vi "Check for Included Angle in Degrees.vi"(5 "coerce output (F)":bool, 7 "output range (-180 to 180)":T1=enum."-180 to 180", 9 "right angle (deg)":dbl, 10 "target angle (deg)":dbl, 11 "left angle (deg)":dbl) -> (1 "in range?":bool, 2 "target angle out (deg)":dbl)   [LabVIEW 2017, in "NI_Robotics Utilities.lvlib"]
doc: "This VI is deprecated. Use <vi.lib>\\Analysis\\coordinate.llb\\Check for Included Angle.vi instead."
uses:
  <vilib>/robotics/Utilities/NI_Robotics Utilities.lvlib
  <vilib>/robotics/Utilities/Angle Range_Degrees.ctl
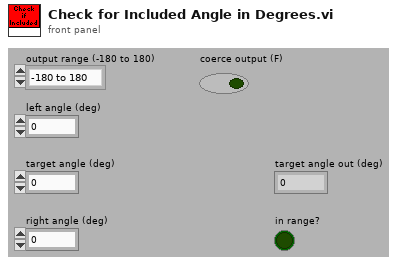
[diagram p1: front panel]
types:
  T1 = typedef "NI_Robotics Utilities.lvlib/Angle Range_Degrees.ctl" = enum16{"none", "-180 to 180", "0 to 360"}
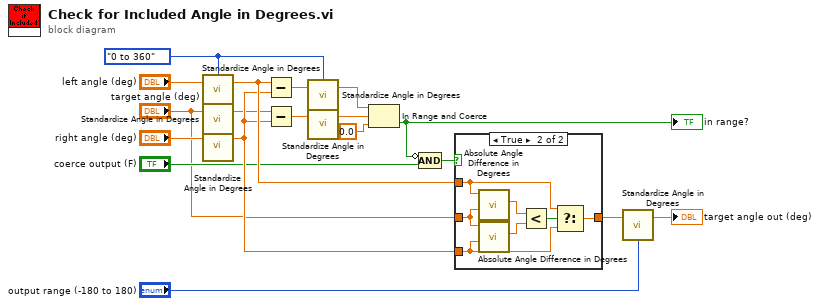
[diagram p0: block diagram]
diagram:
  w13 = Angle_Range_Degrees."0 to 360" ("range (-180 to 180)")
  n1 = call <vilib>:"Standardize Angle in Degrees.vi"("angle in (deg)"="left angle (deg)", "range (-180 to 180)"=w13) -> ("angle out (deg)"=w11:dbl)  [unwired: 3 in]
  n2 = call <vilib>:"Standardize Angle in Degrees.vi"("angle in (deg)"="target angle (deg)", "range (-180 to 180)"=w13) -> ("angle out (deg)"=w1:dbl)  [unwired: 3 in]
  n3 = call <vilib>:"Standardize Angle in Degrees.vi"("angle in (deg)"="right angle (deg)", "range (-180 to 180)"=w13) -> ("angle out (deg)"=w9:dbl)  [unwired: 3 in]
  n4 = Subtract(x=w11, y=w9) -> (x-y=w17:dbl)
  n5 = Subtract(x=w1, y=w9) -> (x-y=w15:dbl)
  n6 = call <vilib>:"Standardize Angle in Degrees.vi"("angle in (deg)"=w17, "range (-180 to 180)"=w13) -> ("angle out (deg)"=w16:dbl)  [unwired: 3 in]
  n7 = call <vilib>:"Standardize Angle in Degrees.vi"("angle in (deg)"=w15, "range (-180 to 180)"=w13) -> ("angle out (deg)"=w14:dbl)  [unwired: 3 in]
  n8 = In Range and Coerce(upper limit=w16, x=w14, lower limit=0.0) -> (In Range?=w7:bool)  [unwired: 1 out]
  "in range?" <- w7
  n9 = Compound Arithmetic op=AND(invert w7, "coerce output (F)") -> (w6:bool)
  n10 = case shown="True" w6 {
    tunnel: w11 -> [_ w22]
    tunnel: "target angle (deg)" -> [w19 w26]
    tunnel: w9 -> [_ w21]
    tunnel: [w19 w20] -> w5
    frame False {
    }
    frame True {
      n11 = call <vilib>:"Absolute Angle Difference in Degrees.vi"("angle 2 (deg)"=w26, "angle 1 (deg)"=w22) -> ("|angle 1 - angle 2| (deg)"=w25:dbl)  [unwired: 9 in]
      n12 = call <vilib>:"Absolute Angle Difference in Degrees.vi"("angle 2 (deg)"=w21, "angle 1 (deg)"=w26) -> ("|angle 1 - angle 2| (deg)"=w24:dbl)  [unwired: 9 in]
      n13 = Less?(x=w25, y=w24) -> (x < y?=w23:bool)
      n14 = Select(t=w22, s=w23, f=w21) -> (s? t:f=w20:dbl)
    }
  }
  n15 = call <vilib>:"Standardize Angle in Degrees.vi"("angle in (deg)"=w5, "range (-180 to 180)"="output range (-180 to 180)") -> ("angle out (deg)"=→"target angle out (deg)":dbl)  [unwired: 3 in]
